vi "Lift Grab Crate State Machine.vi"(0 "State In":T9(ring), 5 "Limit Switches":T13, 7 "Lift Potentiometer":T6, 9 "Gripper Encoder":T2, 11 "From Shift":T1, 12 "Gripper Gains":cluster{"P":dbl, "I":dbl, "D":dbl}) -> (4 "State Out":T9(ring), 6 "Lift Output":dbl, 8 "Gripper Output":dbl, 10 "Done?":bool, 15 "To Shift":T1)   [LabVIEW 2014]
uses:
  <vilib>/Rock Robotics/WPI/Switch/WPI_SwitchDevRef.ctl
  <vilib>/Rock Robotics/SystemInterfaces/DIO/FPGA_DIOChannel.ctl
  <vilib>/Rock Robotics/SystemInterfaces/Typedef/FPGA_TypedefDigitalModule.ctl
  <vilib>/Rock Robotics/SystemInterfaces/Counter/FPGA_CounterCtrSystemIndex.ctl
  <vilib>/Rock Robotics/WPI/Potentiometer/WPI_PotentiometerDevRef.ctl
  <vilib>/Rock Robotics/SystemInterfaces/Typedef/FPGA_TypedefAnalogModule.ctl
  <vilib>/Rock Robotics/SystemInterfaces/AI/FPGA_AIChannel.ctl
  <vilib>/Rock Robotics/WPI/Encoder/WPI_EncoderDevRef.ctl
  <vilib>/Rock Robotics/SystemInterfaces/Encoder/FPGA_EncoderIdx.ctl
  <vilib>/Rock Robotics/WPI/Encoder/WPI_EncoderType.ctl
panel:
  in  "Setpoint":dbl format="%#_13g"
  in  "Setpoint for lowest point":dbl=3.0 format="%#_13g"
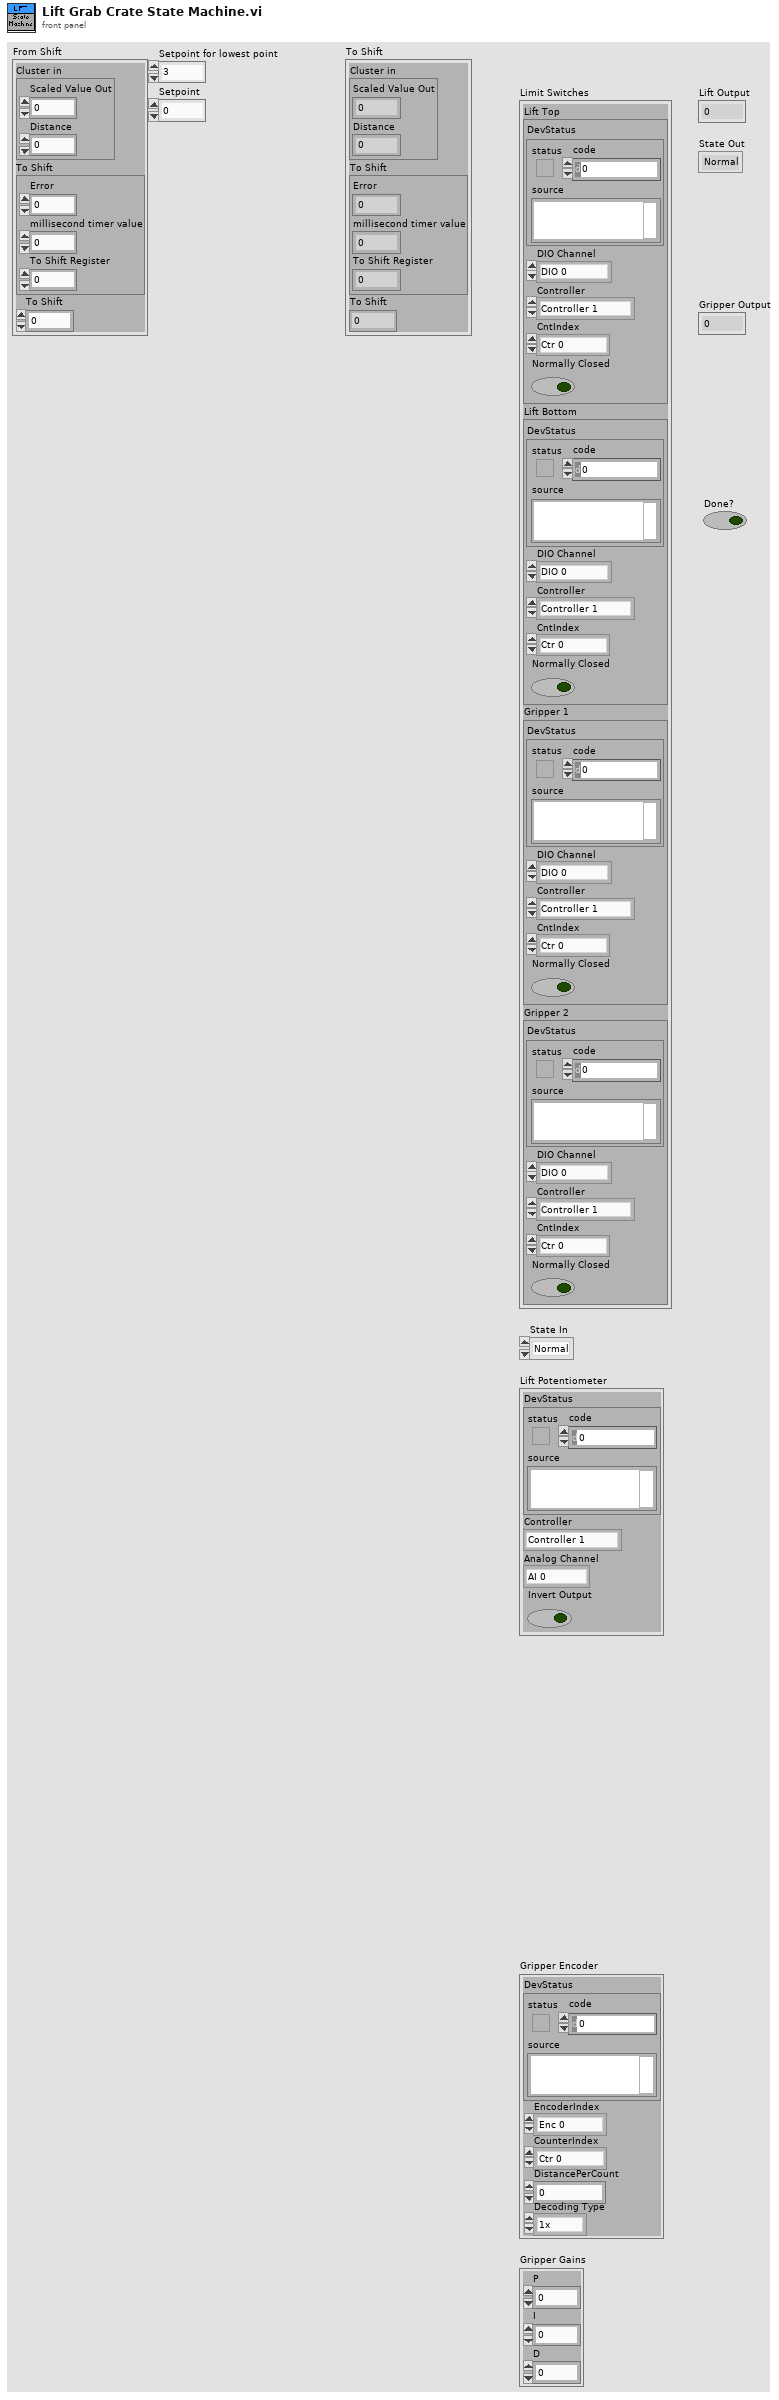
[diagram p1: front panel]
types:
  T1 = cluster{"Cluster in":cluster{"Scaled Value Out":dbl, "Distance":dbl}, "To Shift":cluster{"Error":dbl, "millisecond timer value":u32, "To Shift Register":dbl}, "To Shift":dbl}
  T2 = typedef "WPI_EncoderDevRef.ctl" = cluster{"DevStatus":errorcluster, "EncoderIndex":T3, "CounterIndex":T4, "DistancePerCount":dbl, "Decoding Type":T5}
  T3 = typedef "FPGA_EncoderIdx.ctl" = enum8{"Enc 0", "Enc 1", "Enc 2", "Enc 3", "Enc 4", "Enc 5", "Enc 6", "Enc 7", "Invalid"}
  T4 = typedef "FPGA_CounterCtrSystemIndex.ctl" = enum8{"Ctr 0", "Ctr 1", "Ctr 2", "Ctr 3", "Ctr 4", "Ctr 5", "Ctr 6", "Ctr 7", "Invalid"}
  T5 = typedef "WPI_EncoderType.ctl" = enum16{"1x", "2x", "4x"}
  T6 = typedef "WPI_PotentiometerDevRef.ctl" = cluster{"DevStatus":errorcluster, "Controller":T7, "Analog Channel":T8, "Invert Output":bool}
  T7 = typedef "FPGA_TypedefAnalogModule.ctl" = enum16{"Controller 1"}
  T8 = typedef "FPGA_AIChannel.ctl" = enum8{"AI 0", "AI 1", "AI 2", "AI 3", "AI MXP 0", "AI MXP 1", "AI MXP 2", "AI MXP 3", "Invalid"}
  T9 = enum16{"Normal", "Down/Out", "Down/In", "Up", "Override"}
  T10 = typedef "WPI_SwitchDevRef.ctl" = cluster{"DevStatus":errorcluster, "DIO Channel":T11, "Controller":T12, "CntIndex":T4, "Normally Closed":bool}
  T11 = typedef "FPGA_DIOChannel.ctl" = enum8{"DIO 0", "DIO 1", "DIO 2", "DIO 3", "DIO 4", "DIO 5", "DIO 6", "DIO 7", "DIO 8", "DIO 9", "DIO MXP 0", "DIO MXP 1", "DIO MXP 2", "DIO MXP 3", "DIO MXP 4", "DIO MXP 5", "DIO MXP 6", "DIO MXP 7", "DIO MXP 8", "DIO MXP 9", "DIO MXP 10", "DIO MXP 11", "DIO MXP 12", "DIO MXP 13", "DIO MXP 14", "DIO MXP 15", "Invalid"}
  T12 = typedef "FPGA_TypedefDigitalModule.ctl" = enum16{"Controller 1"}
  T13 = cluster{"Lift Top":T10, "Lift Bottom":T10, "Gripper 1":T10, "Gripper 2":T10}
  T14 = cluster{"Error":dbl, "millisecond timer value":u32, "To Shift Register":dbl}
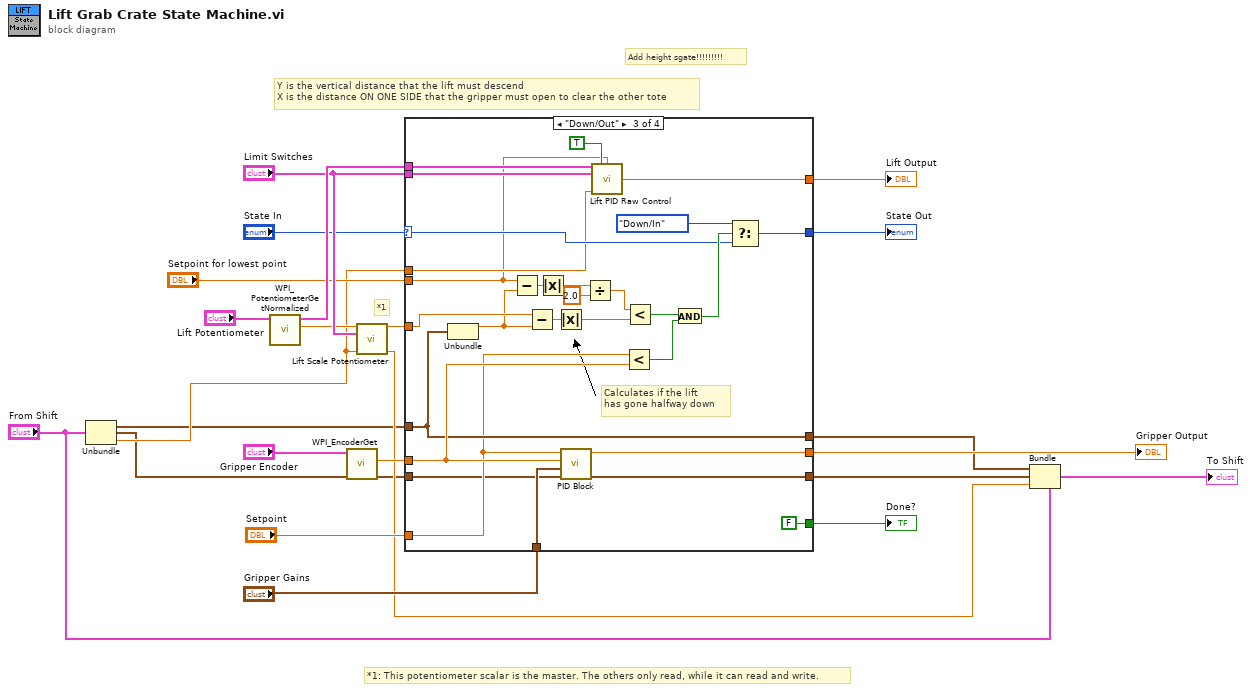
[diagram p0: block diagram]
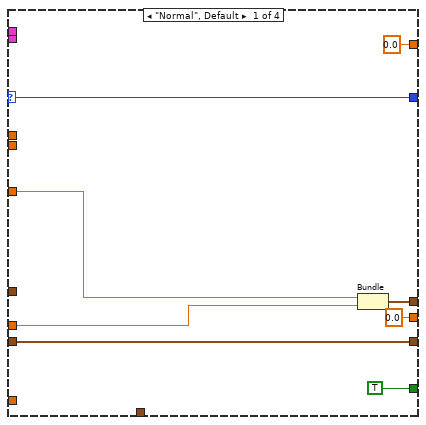
[diagram p2: hidden frame]
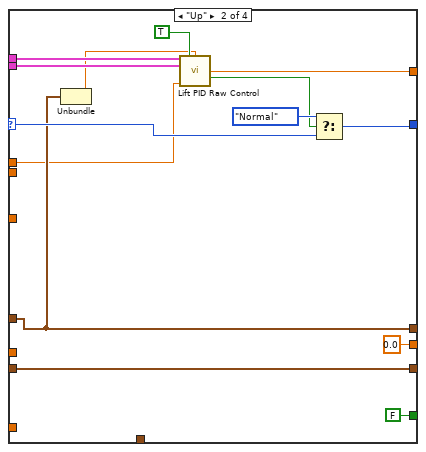
[diagram p3: hidden frame]
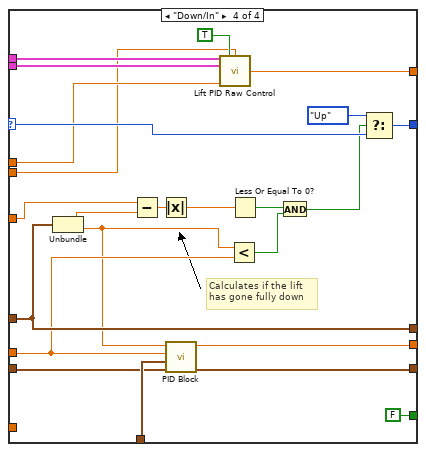
[diagram p4: hidden frame]
diagram:
  # "Add height sgate!!!!!!!!!"
  # "*1: This potentiometer scalar is the master. The others only read, while it can read and write."
  # "*1"
  # "Y is the vertical distance that the lift must descend\nX is the distance ON ONE SIDE that the gripper must open to clear the other tote"
  n1 = Unbundle("From Shift") -> ("Cluster in"=w4:cluster{"Scaled Value Out":dbl, "Distance":dbl}, "To Shift"=w3:T14, "To Shift"=w5:dbl)
  n2 = call <vilib>:"WPI_PotentiometerGetNormalized.vi"("PotDevRef"="Lift Potentiometer") -> ("Normalized Value"=w18:dbl, "PotDevRef"=w21:T6)  [unwired: 8 in, 1 out]
  n3 = call <vilib>:"WPI_EncoderGet.vi"("EncoderDevRef"="Gripper Encoder") -> ("Distance"=w12:dbl)  [unwired: 5 in, 5 out]
  n4 = call "Lift Scale Potentiometer.vi"("Potentiometer In"=w18, "Limit Switches"="Limit Switches", "From Shift"=w5) -> ("Scaled Value Out"=w17:dbl, "To Shift"=w6:dbl)  [unwired: 11 in]
  n5 = case shown="\"Down/Out\"" "State In" {
    selector: "State In" -> [w28 w43 w70 w95]
    tunnel: [w31 w34 w68 w87] -> w8
    tunnel: w17 -> [w30 _ w48 w84]
    tunnel: w12 -> [w29 _ w73 w76]
    tunnel: w4 -> [_ w34 w68 w87]
    tunnel: [w28 w44 w71 w96] -> w11
    tunnel: "Setpoint for lowest point" -> [_ _ w47 w77]
    tunnel: "Setpoint" -> [_ _ w66 _]
    tunnel: [0.0 ("Output") 0.0 ("Output") w64 w86] -> w15
    tunnel: "Gripper Gains" -> [_ _ w63 w89]
    tunnel: w3 -> [w27 w40 w60 w88]
    tunnel: [w27 w40 w59 w85] -> w7
    tunnel: "Limit Switches" -> [_ w36 w56 w81]
    tunnel: w21 -> [_ w37 w57 w80]
    tunnel: w5 -> [_ w32 w55 w79]
    tunnel: [0.0 ("Motor output") w39 w54 w78] -> w22
    tunnel: [TRUE FALSE FALSE FALSE] -> w23
    frame "Normal", Default {
      n6 = Bundle("Scaled Value Out"=w30, "Distance"=w29) -> (w31:cluster{"Scaled Value Out":dbl, "Distance":dbl})  [unwired: 1 in]
    }
    frame "Up" {
      n7 = Unbundle(w34) -> ("Scaled Value Out"=w33:dbl)  [unwired: 1 out]
      n8 = call "Lift PID Raw Control.vi"("Lift Potentionmeter"=w37, "Autonomous?"=TRUE, "Setpoint"=w33, "Limit Switches"=w36, "From Shift"=w32) -> ("Motor output"=w39:dbl, "Tolerable?"=w38:bool)  [unwired: 6 in, 3 out]
      n9 = Select(t=enum16{"Normal", "Down/Out", "Down/In", "Up"}."Normal", s=w38, f=w43) -> (s? t:f=w44:T9)
    }
    frame "Down/Out" {
      # "Calculates if the lift\nhas gone halfway down"
      n10 = Unbundle(w68) -> ("Scaled Value Out"=w46:dbl)  [unwired: 1 out]
      n11 = Subtract(x=w47, y=w46) -> (x-y=w52:dbl)
      n12 = Subtract(x=w48, y=w46) -> (x-y=w67:dbl)
      n13 = Absolute Value(x=w52) -> (abs(x)=w50:dbl)
      n14 = Absolute Value(x=w67) -> (abs(x)=w65:dbl)
      n15 = call "PID Block.vi"("From Shift"=w60, "Gains"=w63, "Position"=w73, "Setpoint"=w66) -> ("To Shift"=w59:T14, "Output"=w64:dbl)  [unwired: 5 in, 1 out]
      n16 = Divide(x=w50, y=2.0) -> (x/y=w51:dbl)
      n17 = call "Lift PID Raw Control.vi"("Lift Potentionmeter"=w57, "Autonomous?"=TRUE, "Setpoint"=w47, "Limit Switches"=w56, "From Shift"=w55) -> ("Motor output"=w54:dbl)  [unwired: 6 in, 4 out]
      n18 = Less?(x=w66, y=w73) -> (x < y?=w61:bool)
      n19 = Less?(x=w51, y=w65) -> (x < y?=w69:bool)
      n20 = And(x=w69, y=w61) -> (x .and. y?=w72:bool)
      n21 = Select(t=T9."Down/In", s=w72, f=w70) -> (s? t:f=w71:T9)
    }
    frame "Down/In" {
      # "Calculates if the lift\nhas gone fully down"
      n22 = Unbundle(w87) -> ("Scaled Value Out"=w90:dbl, "Distance"=w75:dbl)
      n23 = Subtract(x=w84, y=w90) -> (x-y=w93:dbl)
      n24 = Absolute Value(x=w93) -> (abs(x)=w92:dbl)
      n25 = call "PID Block.vi"("From Shift"=w88, "Gains"=w89, "Position"=w76, "Setpoint"=w75) -> ("To Shift"=w85:T14, "Output"=w86:dbl)  [unwired: 5 in, 1 out]
      n26 = call "Lift PID Raw Control.vi"("Lift Potentionmeter"=w80, "Autonomous?"=TRUE, "Setpoint"=w77, "Limit Switches"=w81, "From Shift"=w79) -> ("Motor output"=w78:dbl)  [unwired: 6 in, 4 out]
      n27 = Less?(x=w75, y=w76) -> (x < y?=w91:bool)
      n28 = Less Or Equal To 0?(x=w92) -> (x <= 0?=w94:bool)
      n29 = And(x=w94, y=w91) -> (x .and. y?=w83:bool)
      n30 = Select(t=enum16{"Normal", "Down/Out", "Down/In", "Up"}."Up", s=w83, f=w95) -> (s? t:f=w96:T9)
    }
  }
  "Done?" <- w23
  "Lift Output" <- w22
  "Gripper Output" <- w15
  "State Out" <- w11
  n31 = Bundle(cluster="From Shift", "Cluster in"=w8, "To Shift"=w7, "To Shift"=w6) -> (→"To Shift":T1)
